vi "camera_asynchrone_acquisition-ajg2.vi"() -> ()   [LabVIEW 2020]
uses:
  WaveKit/Controls/Image information.ctl
  WaveKit/Controls/Image general information.ctl
  WaveKit/Controls/Image acquisition information.ctl
  WaveKit/Controls/Point2D.ctl
  WaveKit/Controls/Data alignment enum.ctl
  WaveKit/Classes/Camera/Camera.lvclass
  WaveKit/Classes/CameraSet/CameraSet.lvclass
  WaveKit/Classes/Image/Image.lvclass
panel:
  in  "Path (dialog if empty)":path
  out "Acquisition information":T1={"Image general information"={"Camera serial number"="", "Smearing removed"=FALSE, "Background image removed"=FALSE, "Time Stamp"=timestamp(0 s since 1904-01-01), "Comment"="", "Camera_MAX_Level"=0}, "Acquisition information"={"Exposure duration (us)"=0, "Exposure duration specified (us)"=0, "Gain"=0.0, "Number of summed images"=0, "Trigger type"=""}, "Number of pixels"={"X"=0, "Y"=0}, "Number of bits"=enum."16"}
  in  "Reset error":bool
  out "exposure_duration_us (get)":u32
  in  "exposure_duration_us (set)":u32=1000 min=1
  out "Current error":errorcluster
  out "nb_images (get)":u32=10
  in  "nb_images (set)":u32=1 min=1
  in  "Show camera signal":bool
  in  "Exit":bool
  in  "Stop Acq":bool
  in  "Start Acq":bool
  out "Image Camera":u32[][](graph)
  in  "Configuration file path":path
  # "Acquisition Parameters"
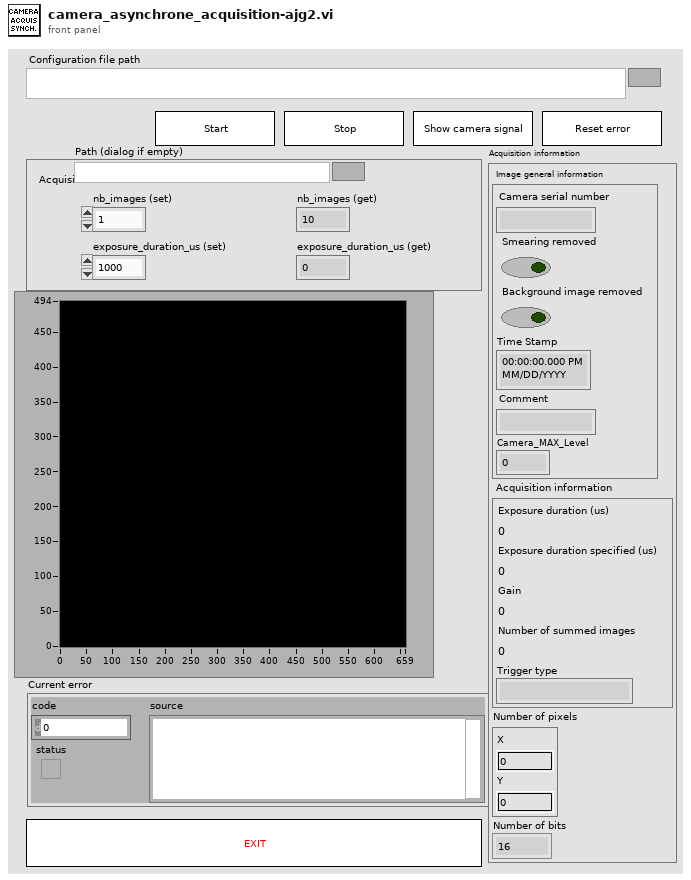
[diagram p1: front panel]
types:
  T1 = typedef "Image information.ctl" = cluster{"Image general information":T2, "Acquisition information":T3, "Number of pixels":T4, "Number of bits":T5}
  T2 = typedef "Image general information.ctl" = cluster{"Camera serial number":string, "Smearing removed":bool, "Background image removed":bool, "Time Stamp":timestamp, "Comment":string, "Camera_MAX_Level":i32}
  T3 = typedef "Image acquisition information.ctl" = cluster{"Exposure duration (us)":i32, "Exposure duration specified (us)":i32, "Gain":sgl, "Number of summed images":i32, "Trigger type":string}
  T4 = typedef "Point2D.ctl" = cluster{"X":u32, "Y":u32}
  T5 = typedef "Data alignment enum.ctl" = enum16{"8", "16", "32"}
  T6 = typedef "CameraSpecifications.ctl" = cluster{"Grabber name":string, "Camera name":string, "Camera sn":string, "Pixels_um":T7, "Maximum level":u32, "Data alignment":T5, "Is signed":bool, "Acquisition start":T4, "Acquisition length":T4, "MaxFrameRate_Hz":sgl, "Chip type":enum16{"Progressive scan", "Frame transfert"}}
  T7 = typedef "General dimensions definition.ctl" = cluster{"Size":T4, "Step":T8}
  T8 = typedef "Point2Df.ctl" = cluster{"X":sgl, "Y":sgl}
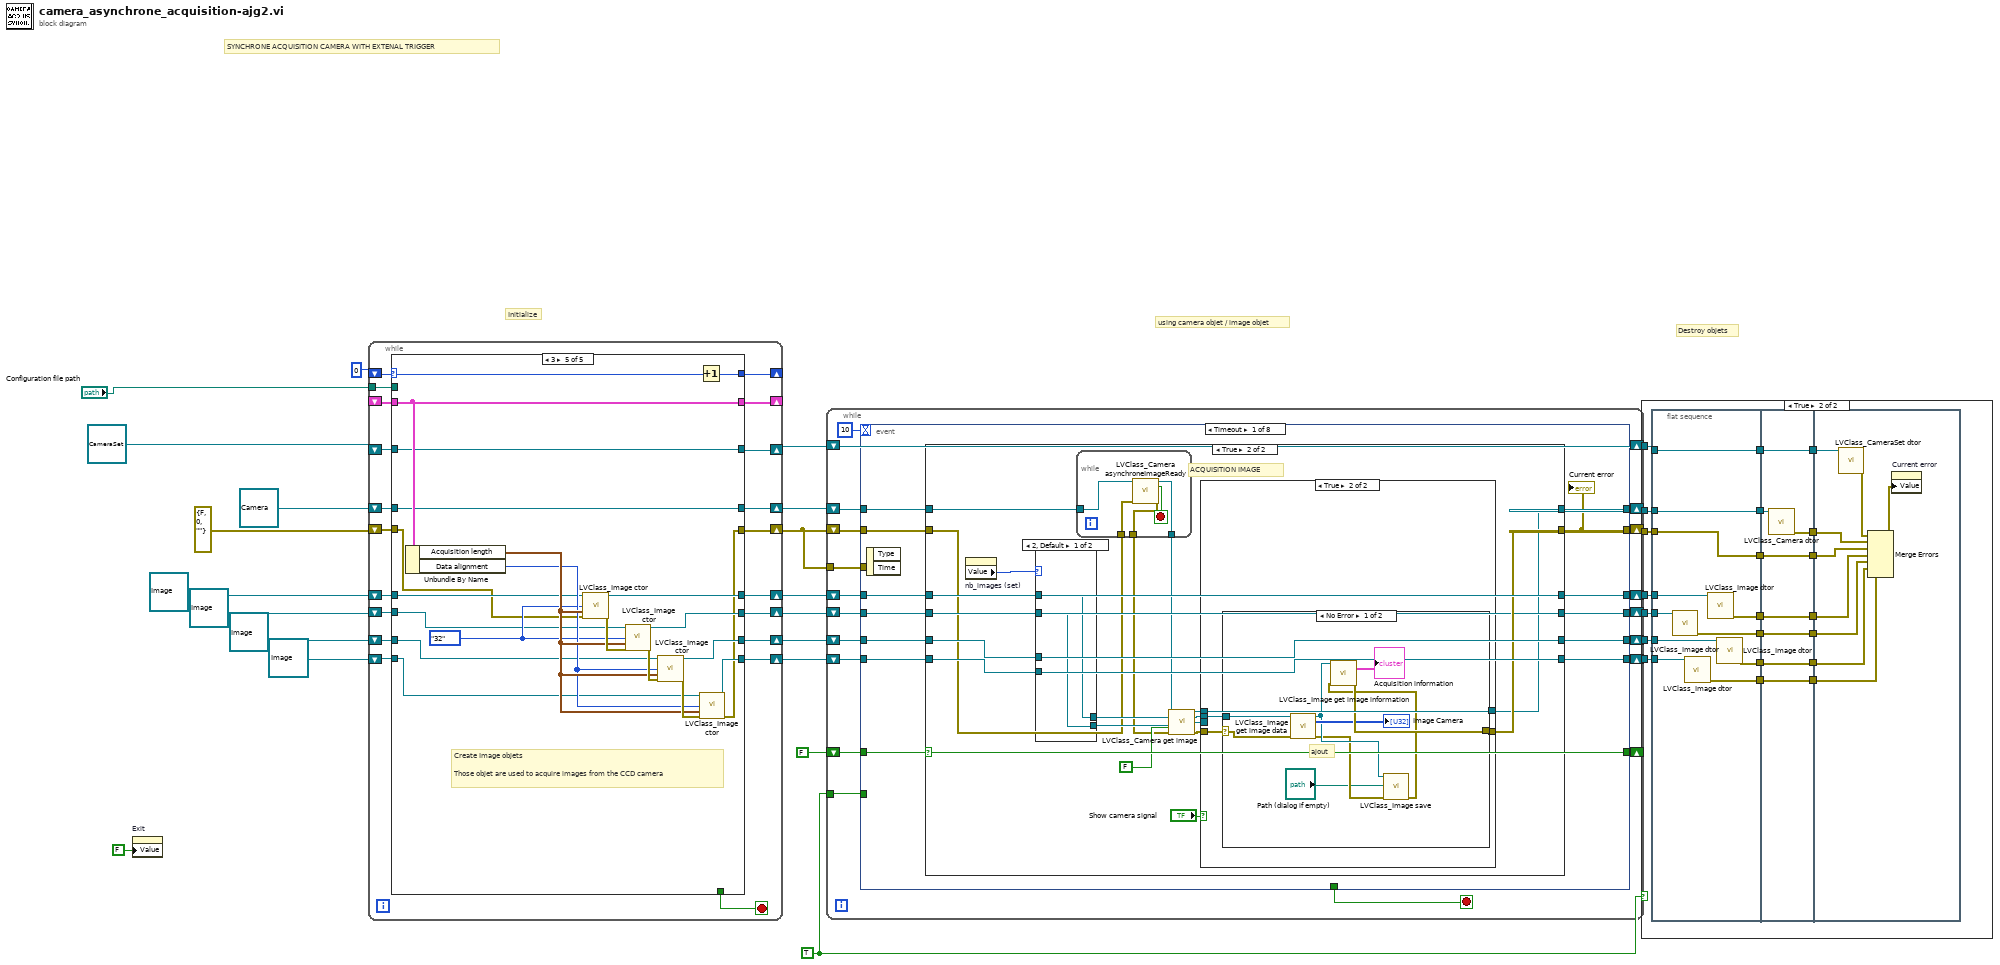
[diagram p0: block diagram]
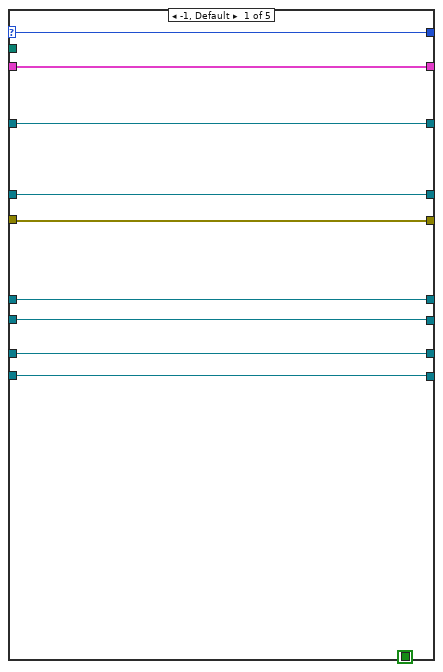
[diagram p2: hidden frame]
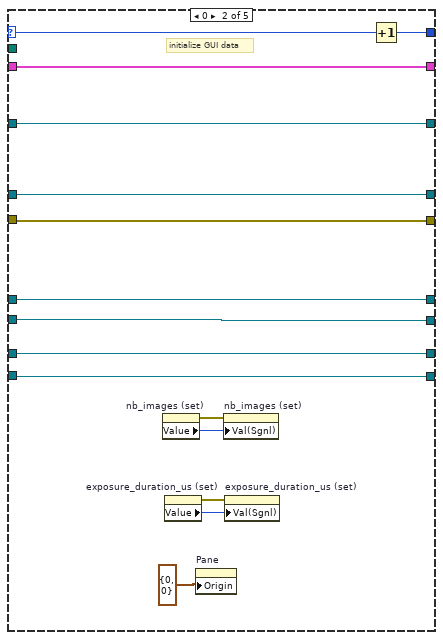
[diagram p3: hidden frame]
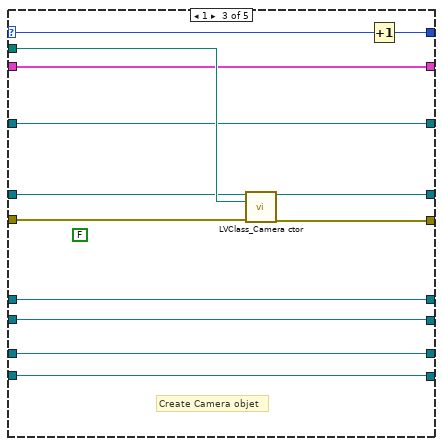
[diagram p4: hidden frame]
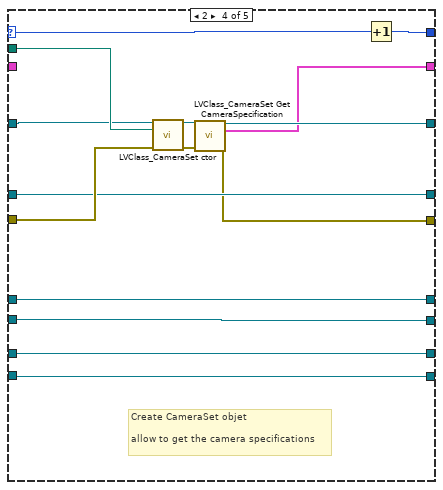
[diagram p5: hidden frame]
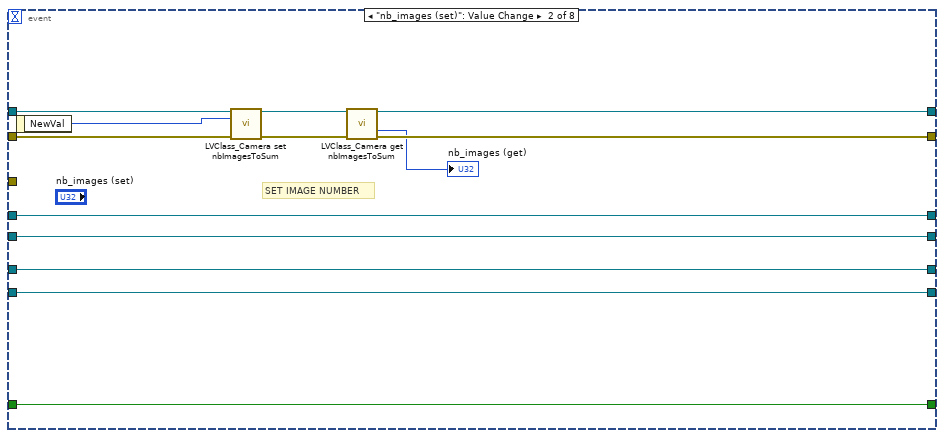
[diagram p11: hidden frame]
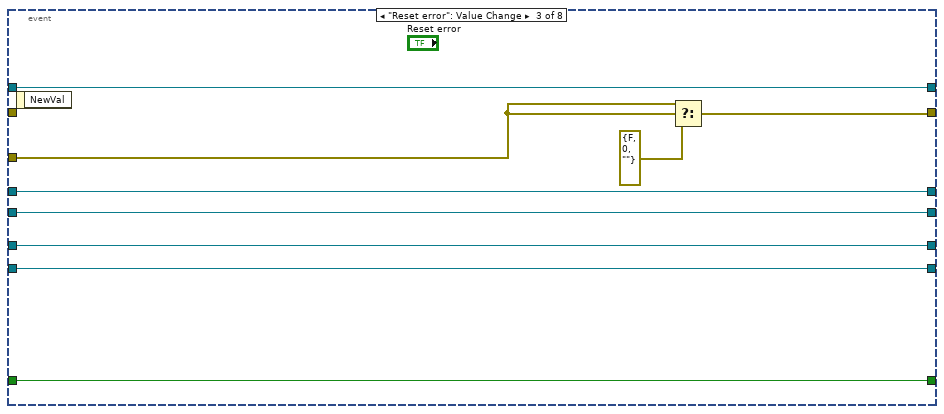
[diagram p12: hidden frame]
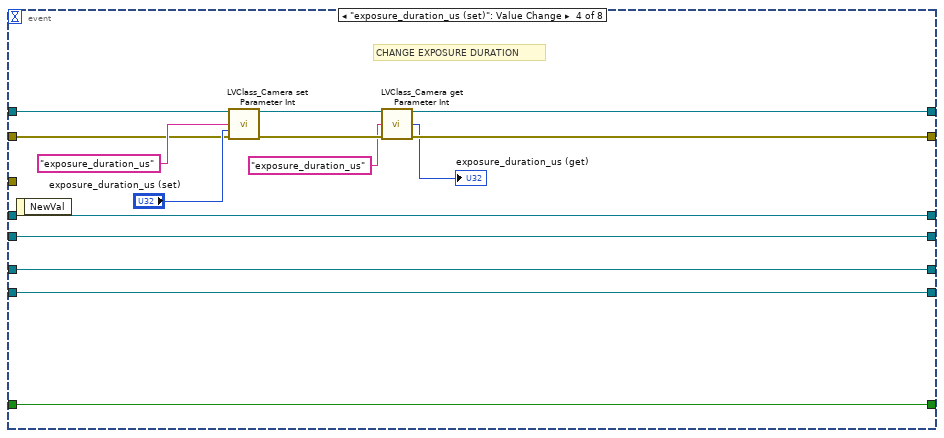
[diagram p13: hidden frame]
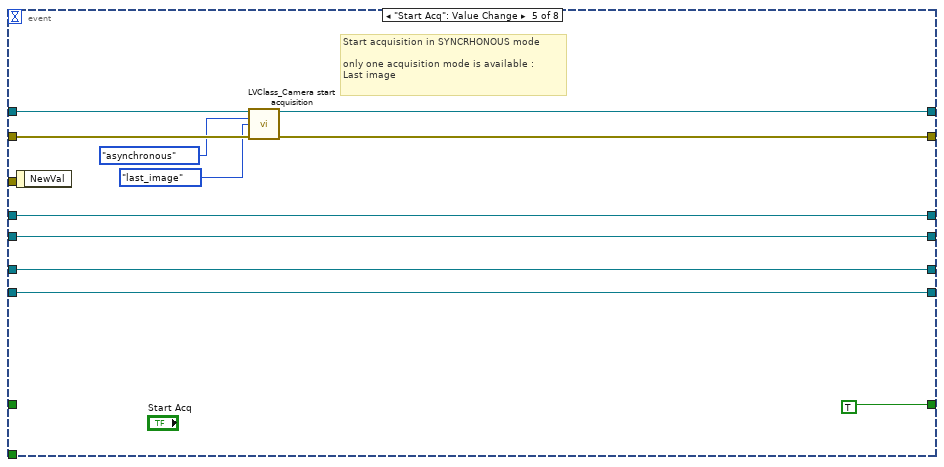
[diagram p14: hidden frame]
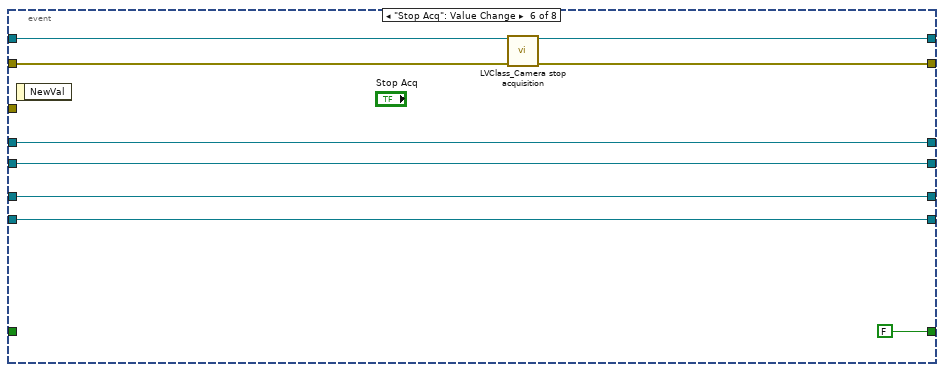
[diagram p15: hidden frame]
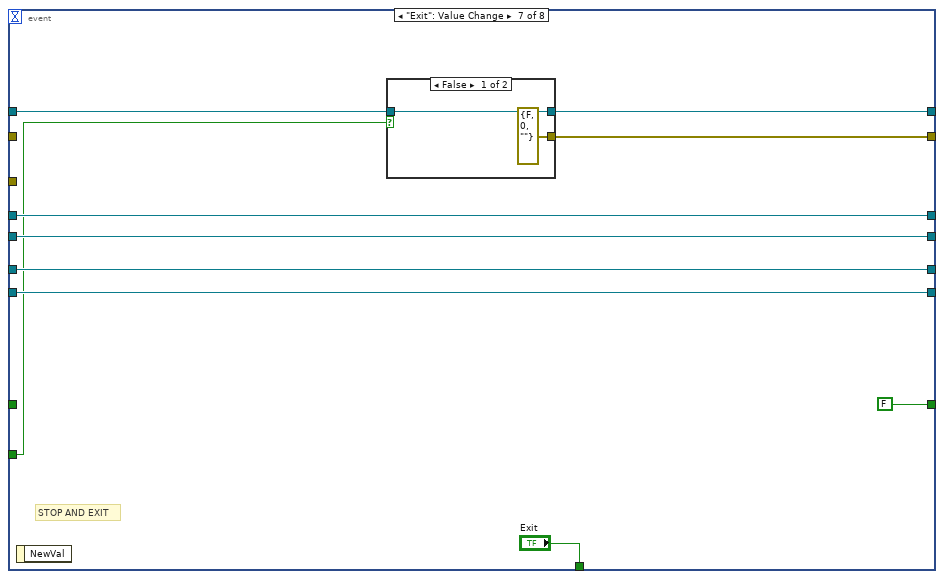
[diagram p16: hidden frame]
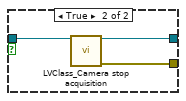
[diagram p17: hidden frame]
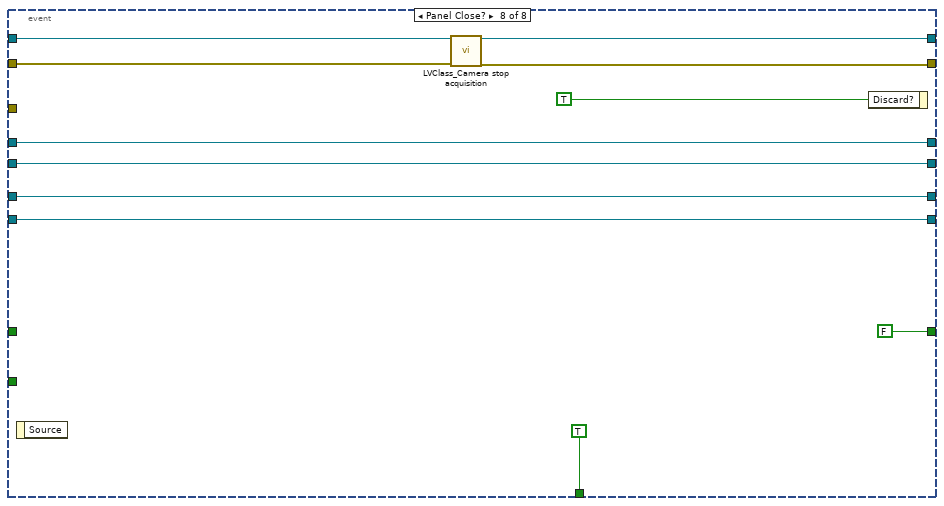
[diagram p18: hidden frame]
diagram:
  w4 = TRUE
  # "Initialize"
  # "Destroy objets"
  # "using camera objet / image objet"
  # "SYNCHRONE ACQUISITION CAMERA WITH EXTENAL TRIGGER"
  n1 = property on="Exit" class="Bool (strict)"("Value"=FALSE ("Exit")) -> ()  [unwired: 2 in, 2 out]
  n2 = while {
    tunnel: "Configuration file path" -> [w44]
    shift-right: [w46] -> w18
    shift-left: refnum<class "Camera.lvclass"> refnum ("Camera.lvclass") -> [w38]
    shift-right: [w28] -> _
    shift-left: 0 -> [w27]
    shift-right: [w45] -> w17
    shift-left: refnum<class "CameraSet.lvclass"> refnum ("CameraSet.lvclass") -> [w37]
    shift-right: [w36] -> _
    shift-left: _ -> [w34]
    shift-right: [w43] -> w16
    shift-left: refnum<class "Image.lvclass"> refnum ("Image in") -> [w35]
    shift-right: [w42] -> w15
    shift-left: refnum<class "Image.lvclass"> refnum ("Image in") -> [w33]
    shift-right: [w41] -> w14
    shift-left: refnum<class "Image.lvclass"> refnum ("Image in") -> [w31]
    shift-right: [w40] -> w13
    shift-left: refnum<class "Image.lvclass"> refnum ("Image in") -> [w32]
    shift-right: [w39] -> w5
    shift-left: errorcluster {"status"=FALSE, "code"=0, "source"=""} ("error out") -> [w29]
    stop <- w30 stop-if-true
    n3 = case shown="3" w27 {
      tunnel: [w56 w58 w84 w92 w107] -> w46
      tunnel: w44 -> [_ _ w83 w96 _]
      tunnel: [w55 w62 w81 w97 w108] -> w45
      tunnel: [w48 w63 w75 w87 w114] -> w43
      tunnel: [w49 w64 w76 w88 w113] -> w42
      tunnel: [w50 w65 w77 w89 w112] -> w41
      tunnel: [w51 w66 w78 w90 w111] -> w40
      tunnel: [w52 w57 w80 w91 w110] -> w39
      selector: w27 -> [w47 w60 w73 w86 w102]
      tunnel: w38 -> [w56 w58 w82 w92 w107]
      tunnel: w37 -> [w55 w62 w81 w95 w108]
      tunnel: [w53 w59 w79 w94 w109] -> w36
      tunnel: w35 -> [w48 w63 w75 w87 w106]
      tunnel: w34 -> [w53 w59 w79 _ w109]
      tunnel: w33 -> [w49 w64 w76 w88 w105]
      tunnel: w32 -> [w51 w66 w78 w90 w104]
      tunnel: w31 -> [w50 w65 w77 w89 w103]
      tunnel: [TRUE _ _ _ _] -> w30
      tunnel: w29 -> [w52 w57 w72 w93 w100]
      tunnel: [w47 w61 w74 w85 w101] -> w28
      frame -1, Default {
      }
      frame 0 {
        # "initialize GUI data"
        n4 = property on="nb_images (set)" class="DigNum (strict)"() -> (error out=w71:errorcluster, "Value"=w70:u32)  [unwired: 2 in, 1 out]
        n5 = property on="exposure_duration_us (set)" class="DigNum (strict)"() -> (error out=w67:errorcluster, "Value"=w69:u32)  [unwired: 2 in, 1 out]
        n6 = property on="Pane" class="Pane"("Origin"=cluster{"Horizontal":i16, "Vertical":i16} {"Horizontal"=0, "Vertical"=0} ("Front Panel Window:Origin")) -> ()  [unwired: 2 in, 2 out]
        n7 = property on="nb_images (set)" class="DigNum (strict)"(error in=w71, "Val(Sgnl)"=w70) -> ()  [unwired: 1 in, 2 out]
        n8 = property on="exposure_duration_us (set)" class="DigNum (strict)"(error in=w67, "Val(Sgnl)"=w69) -> ()  [unwired: 1 in, 2 out]
        n9 = Increment(x=w60) -> (x+1=w61:i32)
      }
      frame 1 {
        (unwired) FALSE ("Acq required")
        # "Create Camera objet"
        n10 = call "LVClass_Camera ctor.vi"("Camera (const)"=w82, "Configuration file path"=w83, "error in (no error)"=w72) -> ("Camera (new)"=w84:refnum<class "Camera.lvclass">, "error out"=w80:errorcluster)  [unwired: 11 in]
        n11 = Increment(x=w73) -> (x+1=w74:i32)
      }
      frame 2 {
        # "Create CameraSet objet\n\nallow to get the camera specifications"
        n12 = call "LVClass_CameraSet ctor.vi"("CameraSet (const)"=w95, "Configuration file path"=w96, "error in (no error)"=w93) -> ("CameraSet (new)"=w99:refnum<class "CameraSet.lvclass">, "error out"=w98:errorcluster)  [unwired: 11 in]
        n13 = call "LVClass_CameraSet Get CameraSpecification.vi"("CameraSet in"=w99, "error in (no error)"=w98) -> ("CameraSet out"=w97:refnum<class "CameraSet.lvclass">, "Camera Config"=w94:T6, "error out"=w91:errorcluster)  [unwired: 11 in]
        n14 = Increment(x=w86) -> (x+1=w85:i32)
      }
      frame 3 {
        w115 = Data_alignment_enum."32" ("Data alignment")
        # "Create Image objets\n\nThose objet are used to acquire images from the CCD camera"
        n15 = Unbundle By Name(w109) -> ("Acquisition length"=w117:T4, "Data alignment"=w116:T5)
        n16 = call "LVClass_Image ctor.vi"("Image (const)"=w106, "Data alignment"=w115, "Size"=w117, "error in (no error)"=w100) -> ("Image (new)"=w114:refnum<class "Image.lvclass">, "error out"=w118:errorcluster)  [unwired: 10 in]
        n17 = call "LVClass_Image ctor.vi"("Image (const)"=w105, "Data alignment"=w115, "Size"=w117, "error in (no error)"=w118) -> ("Image (new)"=w113:refnum<class "Image.lvclass">, "error out"=w119:errorcluster)  [unwired: 10 in]
        n18 = call "LVClass_Image ctor.vi"("Image (const)"=w103, "Data alignment"=w116, "Size"=w117, "error in (no error)"=w119) -> ("Image (new)"=w112:refnum<class "Image.lvclass">, "error out"=w120:errorcluster)  [unwired: 10 in]
        n19 = Increment(x=w102) -> (x+1=w101:i32)
        n20 = call "LVClass_Image ctor.vi"("Image (const)"=w104, "Data alignment"=w116, "Size"=w117, "error in (no error)"=w120) -> ("Image (new)"=w111:refnum<class "Image.lvclass">, "error out"=w110:errorcluster)  [unwired: 10 in]
      }
    }
  }
  n21 = while {
    shift-right: [w136] -> w26
    shift-left: w5 -> [w138]
    shift-right: [w134] -> w25
    shift-left: w18 -> [w135]
    shift-right: [w128] -> w24
    shift-left: w16 -> [w133]
    shift-right: [w127] -> w23
    shift-left: w15 -> [w132]
    shift-right: [w126] -> w22
    shift-left: w14 -> [w131]
    shift-right: [w125] -> w21
    shift-left: w13 -> [w130]
    shift-right: [w124] -> _
    shift-left: FALSE -> [w129]
    shift-right: [w123] -> w20
    shift-left: w17 -> [w123]
    tunnel: w5 -> [w122]
    tunnel: w4 -> [w121]
    stop <- w137 stop-if-true
    n22 = event shown="[0] Timeout" {
      selector: _ -> [_ _ _ _ _ _ _ _]
      dyn-events: _ -> [_ _ _ _ _ _ _ _]
      timeout: 10 -> [_ _ _ _ _ _ _ _]
      tunnel: w138 -> [w144 w214 _ w237 w249 w251 _ w276]
      tunnel: [_ _ _ _ _ _ "Exit" TRUE ("Exit")] -> w137
      tunnel: [w140 w212 w217 w232 w247 w257 w267 w281] -> w136
      tunnel: w135 -> [w149 w213 w219 w236 w250 w258 w268 w283]
      tunnel: [w148 w211 w219 w233 w248 w259 w266 w282] -> w134
      tunnel: w133 -> [w152 w204 w221 w226 w244 w253 w262 w277]
      tunnel: w132 -> [w151 w205 w222 w227 w243 w254 w263 w278]
      tunnel: w131 -> [w150 w206 w223 w228 w242 w255 w264 w279]
      tunnel: w130 -> [w145 w207 w224 w229 w241 w256 w265 w280]
      tunnel: w129 -> [w141 w203 w220 w225 _ _ _ _]
      tunnel: [w147 w204 w221 w226 w244 w253 w262 w277] -> w128
      tunnel: [w146 w205 w222 w227 w243 w254 w263 w278] -> w127
      tunnel: [w143 w206 w223 w228 w242 w255 w264 w279] -> w126
      tunnel: [w142 w207 w224 w229 w241 w256 w265 w280] -> w125
      tunnel: [w141 w203 w220 w225 TRUE FALSE FALSE FALSE] -> w124
      tunnel: w122 -> [_ _ w216 _ _ _ _ _]
      tunnel: w121 -> [_ _ _ _ _ _ w260 _]
      event Timeout {
        n23 = event-data() -> ()  [unwired: 1 in, 2 out]
        n24 = case shown="True" w141 {
          tunnel: [w153 w167] -> w140
          tunnel: w152 -> [w158 w173]
          tunnel: [w158 w173] -> w147
          tunnel: [w154 w164] -> w146
          tunnel: w150 -> [w157 w172]
          tunnel: w145 -> [w156 w171]
          tunnel: [w157 w172] -> w143
          tunnel: [w156 w171] -> w142
          tunnel: w151 -> [w154 w164]
          tunnel: w149 -> [w155 w162]
          tunnel: [w155 w163] -> w148
          tunnel: w144 -> [w153 w160]
          frame False {
          }
          frame True {
            # "ACQUISITION IMAGE"
            n25 = property on="nb_images (set)" class="DigNum (strict)"() -> ("Value"=w174:u32)  [unwired: 2 in, 2 out]
            n26 = case shown="2, Default" w174 {
              tunnel: [w184 w186] -> w175
              tunnel: w164 -> [w183 _]
              tunnel: w173 -> [w184 _]
              tunnel: [w183 w185] -> w170
              tunnel: w172 -> [_ w186]
              tunnel: w171 -> [_ w185]
              frame 2, Default {
              }
              frame 1 {
              }
            }
            n27 = while {
              tunnel: w162 -> [w182]
              tunnel: [w181] -> w161
              tunnel: w160 -> [w179]
              tunnel: [w178] -> w159
              stop <- w180 stop-if-true
              n28 = call "LVClass_Camera asynchroneImageReady.vi"("Camera in"=w182, "error in (no error)"=w179) -> ("Camera out"=w181:refnum<class "Camera.lvclass">, "ready"=w180:bool, "error out"=w178:errorcluster)  [unwired: 11 in]
            }
            n29 = call "LVClass_Camera get image.vi"("Camera in"=w161, "Image"=w175, "Image RAW"=w170, "remove_background"=FALSE, "error in (no error)"=w159) -> ("Camera out"=w177:refnum<class "Camera.lvclass">, "Image (dup)"=w168:refnum<class "Image.lvclass">, "Image (dup) RAW"=w169:refnum<class "Image.lvclass">, "error out"=w165:errorcluster)  [unwired: 7 in]
            n30 = case shown="True" "Show camera signal" {
              tunnel: w177 -> [w188 w189]
              tunnel: w168 -> [_ w190]
              tunnel: w165 -> [w187 w192]
              tunnel: [w188 w189] -> w163
              tunnel: [w187 w191] -> w167
              tunnel: w169 -> [_ _]
              frame False {
              }
              frame True {
                n31 = case shown="No Error" w192 {
                  selector: w192 -> [w201 w202]
                  tunnel: [w200 w202] -> w191
                  tunnel: w190 -> [w199 _]
                  frame No Error {
                    # "ajout"
                    n32 = call "LVClass_Image get image data.vi"("Image in"=w199, "error in (no error)"=w201) -> ("Image out"=w196:refnum<class "Image.lvclass">, "Image data out"=→"Image Camera":u32[][], "error out"=w195:errorcluster)  [unwired: 11 in]
                    n33 = call "LVClass_Image save.vi"("Image in"=w196, "Path (dialog if empty)"="Path (dialog if empty)", "error in (no error)"=w195) -> ("error out"=w194:errorcluster)  [unwired: 11 in, 1 out]
                    n34 = call "LVClass_Image get image information.vi"("Image in"=w196, "error in (no error)"=w194) -> ("Acquisition information"=→"Acquisition information":T1, "error out"=w200:errorcluster)  [unwired: 11 in, 1 out]
                  }
                  frame Error {
                  }
                }
              }
            }
          }
        }
        "Current error" <- w140
      }
      event "nb_images (set)": Value Change {
        # "SET IMAGE NUMBER"
        n35 = event-data() -> ("NewVal"=w215:u32)  [unwired: 1 in]
        n36 = call "LVClass_Camera set nbImagesToSum.vi"("Camera in"=w213, "nb_image"=w215, "error in (no error)"=w214) -> ("Camera out"=w210:refnum<class "Camera.lvclass">, "error out"=w209:errorcluster)  [unwired: 11 in]
        n37 = call "LVClass_Camera get nbImagesToSum.vi"("Camera in"=w210, "error in (no error)"=w209) -> ("Camera out"=w211:refnum<class "Camera.lvclass">, "nb_image"=→"nb_images (get)":u32, "error out"=w212:errorcluster)  [unwired: 11 in]
      }
      event "Reset error": Value Change {
        n38 = event-data() -> ()  [unwired: 1 in, 1 out]
        n39 = Select(t=w216, s=w216, f=errorcluster {"status"=FALSE, "code"=0, "source"=""} ("error out")) -> (s? t:f=w217:errorcluster)
      }
      event "exposure_duration_us (set)": Value Change {
        # "CHANGE EXPOSURE DURATION"
        n40 = event-data() -> ()  [unwired: 1 in, 1 out]
        n41 = call "LVClass_Camera set Parameter Int.vi"("Camera in"=w236, "parameter_name"="exposure_duration_us", "value"="exposure_duration_us (set)", "error in (no error)"=w237) -> ("Camera out"=w235:refnum<class "Camera.lvclass">, "error out"=w234:errorcluster)  [unwired: 10 in]
        n42 = call "LVClass_Camera get Parameter Int.vi"("Camera in"=w235, "parameter_name"="exposure_duration_us", "error in (no error)"=w234) -> ("Camera out"=w233:refnum<class "Camera.lvclass">, "value"=→"exposure_duration_us (get)":i32, "error out"=w232:errorcluster)  [unwired: 10 in]
      }
      event "Start Acq": Value Change {
        # "Start acquisition in SYNCRHONOUS mode\n\nonly one acquisition mode is available :\nLast image"
        n43 = event-data() -> ()  [unwired: 1 in, 1 out]
        n44 = call "LVClass_Camera start acquisition.vi"("Camera in"=w250, "synchronisation_mode"=enum16{"synchronous", "asynchronous"}."asynchronous", "acquisition_mode"=enum16{"last_image", "new_image"}."last_image", "error in (no error)"=w249) -> ("Camera out"=w248:refnum<class "Camera.lvclass">, "error out"=w247:errorcluster)  [unwired: 10 in]
      }
      event "Stop Acq": Value Change {
        n45 = event-data() -> ()  [unwired: 1 in, 1 out]
        n46 = call "LVClass_Camera stop acquisition.vi"("Camera in"=w258, "error in (no error)"=w251) -> ("Camera out"=w259:refnum<class "Camera.lvclass">, "error out"=w257:errorcluster)  [unwired: 12 in]
      }
      event "Exit": Value Change {
        # "STOP AND EXIT"
        n47 = event-data() -> ()  [unwired: 1 in, 1 out]
        n48 = case shown="False" w260 {
          tunnel: w268 -> [w271 w274]
          tunnel: [errorcluster {"status"=FALSE, "code"=0, "source"=""} ("error out") w273] -> w267
          tunnel: [w271 w272] -> w266
          frame False {
          }
          frame True {
            n49 = call "LVClass_Camera stop acquisition.vi"("Camera in"=w274) -> ("Camera out"=w272:refnum<class "Camera.lvclass">, "error out"=w273:errorcluster)  [unwired: 13 in]
          }
        }
      }
      event Panel Close? {
        n50 = event-data() -> ()  [unwired: 1 in, 1 out]
        n51 = call "LVClass_Camera stop acquisition.vi"("Camera in"=w283, "error in (no error)"=w276) -> ("Camera out"=w282:refnum<class "Camera.lvclass">, "error out"=w281:errorcluster)  [unwired: 12 in]
        n52 = event-data("Discard?"=TRUE) -> ()  [unwired: 1 in, 1 out]
      }
    }
  }
  n53 = case shown="True" w4 {
    tunnel: w26 -> [_ w292]
    tunnel: w25 -> [_ w291]
    tunnel: w24 -> [_ w290]
    tunnel: w23 -> [_ w289]
    tunnel: w22 -> [_ w288]
    tunnel: w21 -> [_ w287]
    tunnel: w20 -> [_ w286]
    frame False {
    }
    frame True {
      n54 = flat-sequence {
        tunnel: w291 -> [w317]
        tunnel: w292 -> [w315]
        tunnel: [w317] -> w306
        tunnel: w286 -> [w316]
        tunnel: [w316] -> w305
        tunnel: [w315] -> w304
        tunnel: w290 -> [w314]
        tunnel: w289 -> [w313]
        tunnel: w288 -> [w312]
        tunnel: w287 -> [w311]
        tunnel: [w310] -> w303
        tunnel: [w309] -> w302
        tunnel: [w308] -> w301
        tunnel: [w307] -> w300
        tunnel: w306 -> [w325]
        tunnel: w305 -> [w324]
        tunnel: w304 -> [w322]
        tunnel: [w324] -> w299
        tunnel: [w323] -> w298
        tunnel: [w322] -> w297
        tunnel: w303 -> [w321]
        tunnel: [w321] -> w296
        tunnel: w302 -> [w320]
        tunnel: [w320] -> w295
        tunnel: w301 -> [w319]
        tunnel: [w319] -> w294
        tunnel: w300 -> [w318]
        tunnel: [w318] -> w293
        tunnel: w299 -> [w334]
        tunnel: w298 -> [w332]
        tunnel: w297 -> [w331]
        tunnel: w296 -> [w330]
        tunnel: w295 -> [w329]
        tunnel: w294 -> [w328]
        tunnel: w293 -> [w327]
        frame #0 {
          n55 = call "LVClass_Image dtor.vi"("Image in"=w313) -> ("error out"=w309:errorcluster)  [unwired: 13 in, 1 out]
          n56 = call "LVClass_Image dtor.vi"("Image in"=w311) -> ("error out"=w307:errorcluster)  [unwired: 13 in, 1 out]
          n57 = call "LVClass_Image dtor.vi"("Image in"=w314) -> ("error out"=w310:errorcluster)  [unwired: 13 in, 1 out]
          n58 = call "LVClass_Image dtor.vi"("Image in"=w312) -> ("error out"=w308:errorcluster)  [unwired: 13 in, 1 out]
        }
        frame #1 {
          n59 = call "LVClass_Camera dtor.vi"("Camera in"=w325) -> ("error out"=w323:errorcluster)  [unwired: 13 in, 1 out]
        }
        frame #2 {
          n60 = call "LVClass_CameraSet dtor.vi"("CameraSet in"=w334) -> ("error out"=w333:errorcluster)  [unwired: 13 in, 1 out]
          n61 = Merge Errors(w333, w332, w331, w330, w329, w328, w327) -> (w326:errorcluster)
          n62 = property on="Current error" class="Clust (strict)"("Value"=w326) -> ()  [unwired: 2 in, 2 out]
        }
      }
    }
  }
